vi "CRISValueRelay.vi"() -> ()   [LabVIEW 2013]
panel:
  in  "WL OOR":bool
  in  "PSB Cycle Number":i32
  in  "Linewidth Readout":dbl
  in  "Power Readout":dbl
  out "WS7 Pattern2 Data":dbl[](graph)
  out "Scan Number":i32
  in  "RILIS OK":bool
  out "CRIS OK":bool
  in  "Thin Readback":i32
  out "Thin Set":i32
  in  "Thick Readback":i32
  out "Thick Set":i32
  in  "Start supercycle":bool
  in  "Bunches in supercycle":i32
  in  "Bunches for HRS":i32
  in  "Power CRIS":dbl format="%#_10g"
  in  "Wavenumber CRIS":dbl format="%#_7g"
  in  "Update Rate (milliseconds)":u32=10
  out "Loop Counter":i32
  in  "Stop Button":bool
  out "isNew":bool
  in  "isOK":bool
  out "waveSet":dbl format="%.4g"
  in  "waveReadback":dbl format="%.4g"
  # "\\\\PCCRIS6\\Narrow Band TiSa Scanner Shared Variables\\isOK"
  # "\\\\PCCRIS6\\Narrow Band TiSa Scanner Shared Variables\\isOK"
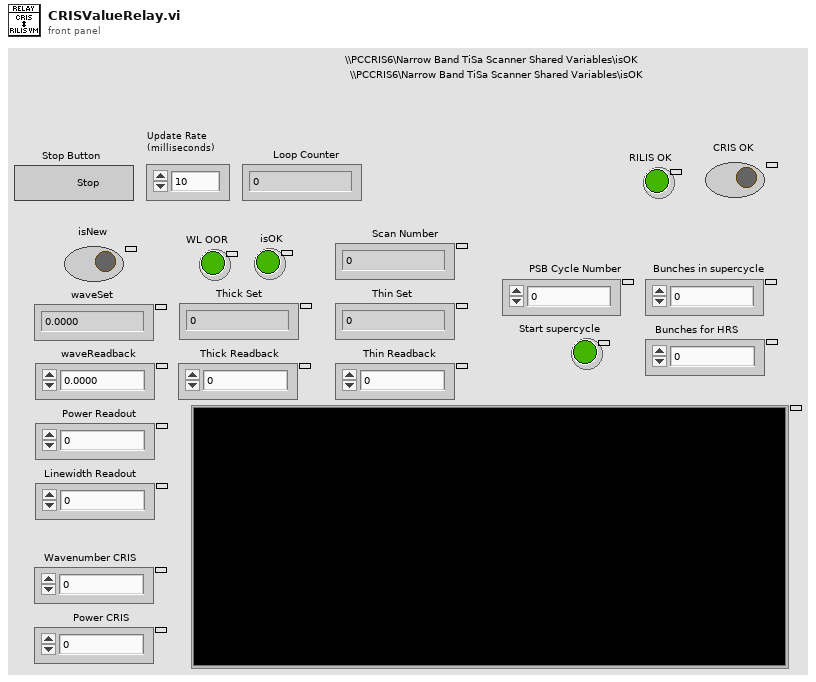
[diagram p1: front panel]
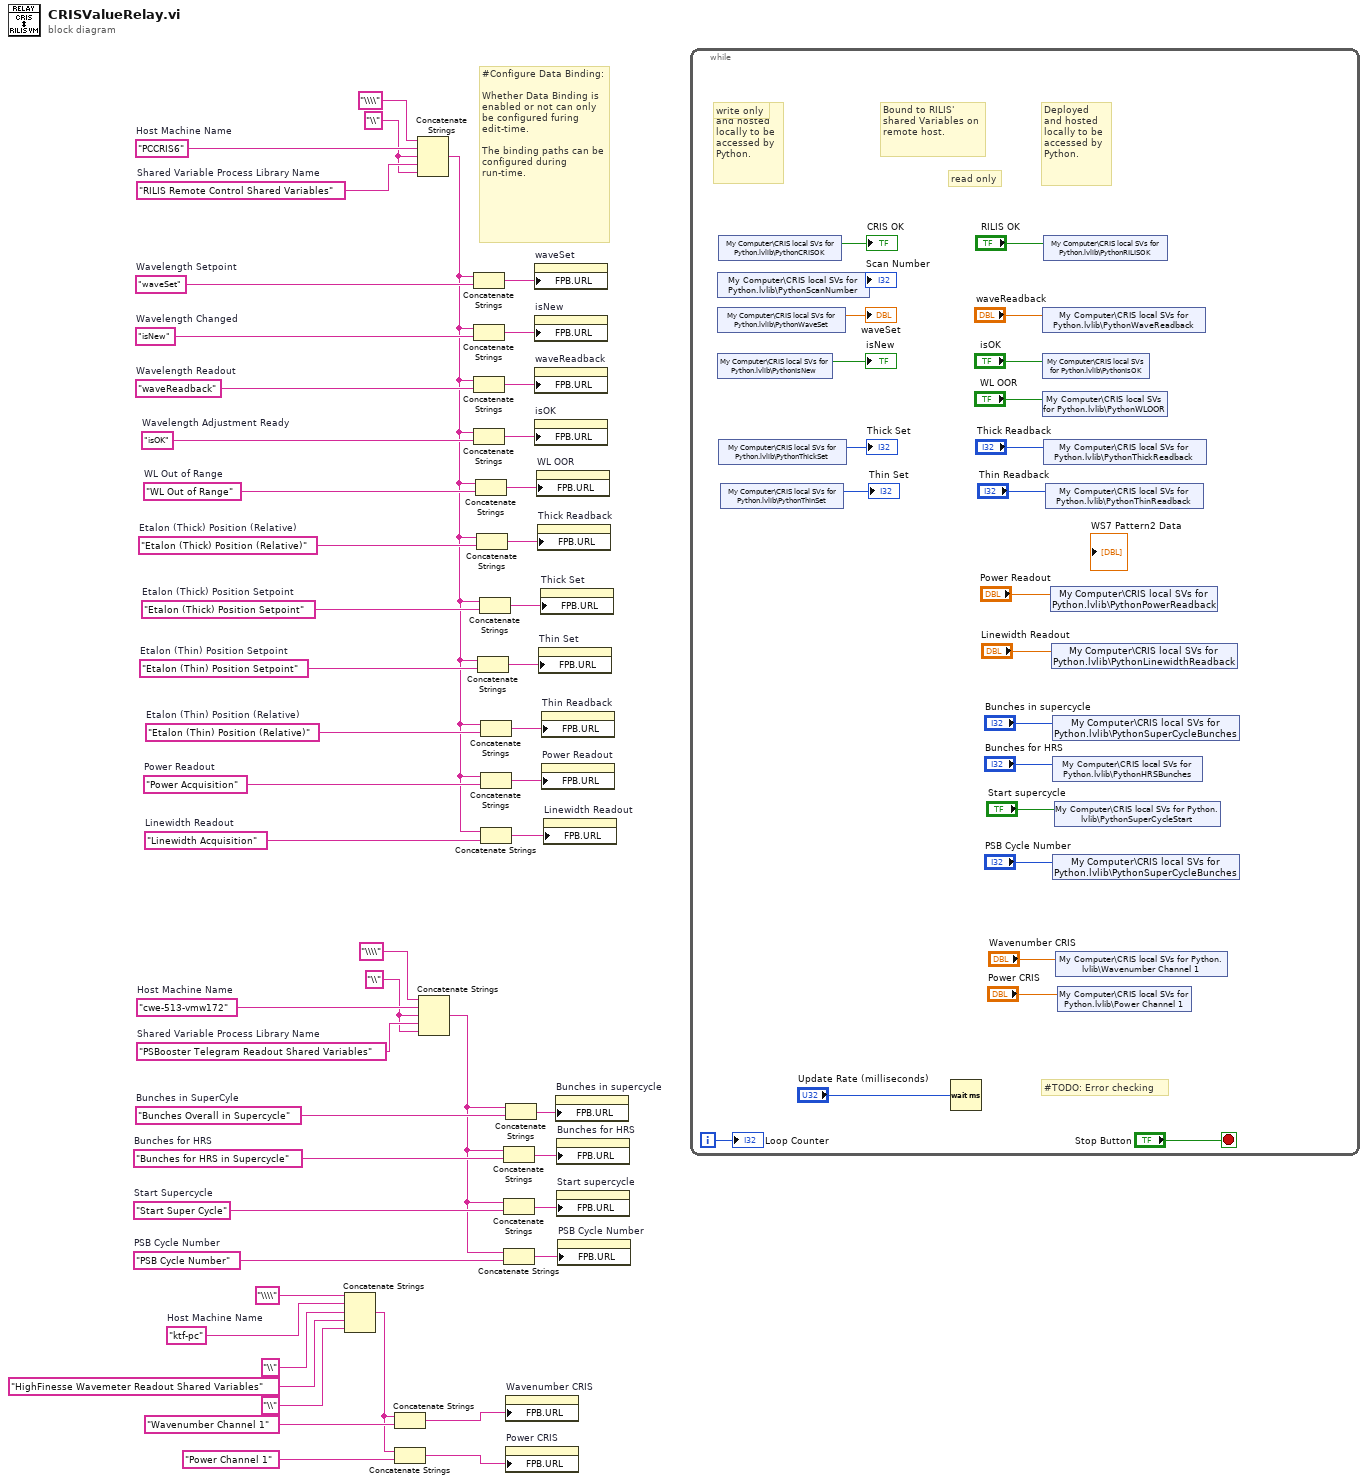
[diagram p0: block diagram]
diagram:
  w2 = "WL Out of Range"  # WL Out of Range
  w7 = "PSB Cycle Number"  # PSB Cycle Number
  w9 = "Linewidth Acquisition"  # Linewidth Readout
  w11 = "Power Acquisition"  # Power Readout
  w4 = "Etalon (Thin) Position Setpoint"  # Etalon (Thin) Position Setpoint
  w5 = "Etalon (Thin) Position (Relative)"  # Etalon (Thin) Position (Relative)
  w15 = "Etalon (Thick) Position Setpoint"  # Etalon (Thick) Position Setpoint
  w17 = "Etalon (Thick) Position (Relative)"  # Etalon (Thick) Position (Relative)
  w20 = "Start Super Cycle"  # Start Supercycle
  w22 = "Bunches Overall in Supercycle"  # Bunches in SuperCyle
  w23 = "\\"
  w24 = "PSBooster Telegram Readout Shared Variables"  # Shared Variable Process Library Name
  w25 = "cwe-513-vmw172"  # Host Machine Name
  w28 = "Bunches for HRS in Supercycle"  # Bunches for HRS
  w32 = "ktf-pc"  # Host Machine Name
  w47 = "\\"
  w46 = "waveSet"  # Wavelength Setpoint
  w40 = "waveReadback"  # Wavelength Readout
  w39 = "isOK"  # Wavelength Adjustment Ready
  w48 = "RILIS Remote Control Shared Variables"  # Shared Variable Process Library Name
  w41 = "isNew"  # Wavelength Changed
  w49 = "PCCRIS6"  # Host Machine Name
  # "#Configure Data Binding:\n\nWhether Data Binding is enabled or not can only be configured furing edit-time.\n\nThe binding paths can be configured during run-time."
  n1 = Concatenate Strings("\\\\", w32, "\\", "HighFinesse Wavemeter Readout Shared Variables", "\\") -> (w29:string)
  n2 = Concatenate Strings(w29, "Wavenumber Channel 1") -> (w31:string)
  n3 = Concatenate Strings(w29, "Power Channel 1") -> (w30:string)
  n4 = Concatenate Strings("\\\\", w49, w47, w48, w47) -> (w1:string)
  n5 = Concatenate Strings("\\\\", w25, w23, w24, w23) -> (w6:string)
  n6 = Concatenate Strings(w1, w46) -> (w45:string)
  n7 = Concatenate Strings(w1, w41) -> (w44:string)
  n8 = Concatenate Strings(w1, w40) -> (w43:string)
  n9 = Concatenate Strings(w1, w39) -> (w42:string)
  n10 = Concatenate Strings(w1, w2) -> (w3:string)
  n11 = Concatenate Strings(w1, w17) -> (w18:string)
  n12 = Concatenate Strings(w1, w4) -> (w14:string)
  n13 = Concatenate Strings(w1, w15) -> (w16:string)
  n14 = Concatenate Strings(w1, w5) -> (w13:string)
  n15 = Concatenate Strings(w1, w11) -> (w12:string)
  n16 = Concatenate Strings(w1, w9) -> (w10:string)
  n17 = Concatenate Strings(w6, w28) -> (w27:string)
  n18 = Concatenate Strings(w6, w20) -> (w19:string)
  n19 = Concatenate Strings(w6, w7) -> (w8:string)
  n20 = Concatenate Strings(w6, w22) -> (w21:string)
  n21 = property on="Wavenumber CRIS" class="DigNum (strict)"("FPB.URL"=w31) -> ()  [unwired: 2 in, 2 out]
  n22 = property on="Power CRIS" class="DigNum (strict)"("FPB.URL"=w30) -> ()  [unwired: 2 in, 2 out]
  n23 = property on="waveSet" class="DigNum (strict)"("FPB.URL"=w45) -> ()  [unwired: 2 in, 2 out]
  n24 = property on="isNew" class="Bool (strict)"("FPB.URL"=w44) -> ()  [unwired: 2 in, 2 out]
  n25 = property on="waveReadback" class="DigNum (strict)"("FPB.URL"=w43) -> ()  [unwired: 2 in, 2 out]
  n26 = property on="isOK" class="Bool (strict)"("FPB.URL"=w42) -> ()  [unwired: 2 in, 2 out]
  n27 = property on="WL OOR" class="Bool (strict)"("FPB.URL"=w3) -> ()  [unwired: 2 in, 2 out]
  n28 = property on="Thick Readback" class="DigNum (strict)"("FPB.URL"=w18) -> ()  [unwired: 2 in, 2 out]
  n29 = property on="Thin Set" class="DigNum (strict)"("FPB.URL"=w14) -> ()  [unwired: 2 in, 2 out]
  n30 = property on="Thick Set" class="DigNum (strict)"("FPB.URL"=w16) -> ()  [unwired: 2 in, 2 out]
  n31 = property on="Thin Readback" class="DigNum (strict)"("FPB.URL"=w13) -> ()  [unwired: 2 in, 2 out]
  n32 = property on="Power Readout" class="DigNum (strict)"("FPB.URL"=w12) -> ()  [unwired: 2 in, 2 out]
  n33 = property on="Linewidth Readout" class="DigNum (strict)"("FPB.URL"=w10) -> ()  [unwired: 2 in, 2 out]
  n34 = property on="Bunches in supercycle" class="DigNum (strict)"("FPB.URL"=w21) -> ()  [unwired: 2 in, 2 out]
  n35 = property on="Bunches for HRS" class="DigNum (strict)"("FPB.URL"=w27) -> ()  [unwired: 2 in, 2 out]
  n36 = property on="Start supercycle" class="Bool (strict)"("FPB.URL"=w19) -> ()  [unwired: 2 in, 2 out]
  n37 = property on="PSB Cycle Number" class="DigNum (strict)"("FPB.URL"=w8) -> ()  [unwired: 2 in, 2 out]
  n38 = while {
    i -> [w72]
    stop <- "Stop Button" stop-if-true
    # "#TODO: Error checking"
    # "Deployed and hosted locally to be accessed by Python."
    # "Deployed and hosted locally to be accessed by Python."
    # "read only"
    # "write only"
    # "Bound to RILIS' shared Variables on remote host."
    n39 = shared-variable "My Computer\\CRIS local SVs for Python.lvlib\\PythonScanNumber"() -> (→"Scan Number":i32)  [unwired: 1 in, 1 out]
    n40 = shared-variable "My Computer\\CRIS local SVs for Python.lvlib\\PythonWaveSet"() -> (→"waveSet":dbl)  [unwired: 1 in, 1 out]
    n41 = shared-variable "My Computer\\CRIS local SVs for Python.lvlib\\PythonIsNew"() -> (→"isNew":bool)  [unwired: 1 in, 1 out]
    n42 = shared-variable "My Computer\\CRIS local SVs for Python.lvlib\\PythonCRISOK"() -> (→"CRIS OK":bool)  [unwired: 1 in, 1 out]
    n43 = shared-variable "My Computer\\CRIS local SVs for Python.lvlib\\PythonThickSet"() -> (→"Thick Set":i32)  [unwired: 1 in, 1 out]
    n44 = shared-variable "My Computer\\CRIS local SVs for Python.lvlib\\PythonThinSet"() -> (→"Thin Set":i32)  [unwired: 1 in, 1 out]
    n45 = Wait (ms)(milliseconds to wait="Update Rate (milliseconds)") -> ()  [unwired: 1 out]
    n46 = shared-variable "My Computer\\CRIS local SVs for Python.lvlib\\PythonWaveReadback"("waveReadback") -> ()  [unwired: 1 in, 1 out]
    n47 = shared-variable "My Computer\\CRIS local SVs for Python.lvlib\\PythonIsOK"("isOK") -> ()  [unwired: 1 in, 1 out]
    n48 = shared-variable "My Computer\\CRIS local SVs for Python.lvlib\\PythonWLOOR"("WL OOR") -> ()  [unwired: 1 in, 1 out]
    n49 = shared-variable "My Computer\\CRIS local SVs for Python.lvlib\\PythonRILISOK"("RILIS OK") -> ()  [unwired: 1 in, 1 out]
    n50 = shared-variable "My Computer\\CRIS local SVs for Python.lvlib\\PythonThickReadback"("Thick Readback") -> ()  [unwired: 1 in, 1 out]
    n51 = shared-variable "My Computer\\CRIS local SVs for Python.lvlib\\PythonThinReadback"("Thin Readback") -> ()  [unwired: 1 in, 1 out]
    n52 = shared-variable "My Computer\\CRIS local SVs for Python.lvlib\\PythonPowerReadback"("Power Readout") -> ()  [unwired: 1 in, 1 out]
    n53 = shared-variable "My Computer\\CRIS local SVs for Python.lvlib\\PythonLinewidthReadback"("Linewidth Readout") -> ()  [unwired: 1 in, 1 out]
    n54 = shared-variable "My Computer\\CRIS local SVs for Python.lvlib\\PythonSuperCycleBunches"("Bunches in supercycle") -> ()  [unwired: 1 in, 1 out]
    n55 = shared-variable "My Computer\\CRIS local SVs for Python.lvlib\\PythonHRSBunches"("Bunches for HRS") -> ()  [unwired: 1 in, 1 out]
    n56 = shared-variable "My Computer\\CRIS local SVs for Python.lvlib\\PythonSuperCycleBunches"("PSB Cycle Number") -> ()  [unwired: 1 in, 1 out]
    n57 = shared-variable "My Computer\\CRIS local SVs for Python.lvlib\\PythonSuperCycleStart"("Start supercycle") -> ()  [unwired: 1 in, 1 out]
    n58 = shared-variable "My Computer\\CRIS local SVs for Python.lvlib\\Wavenumber Channel 1"("Wavenumber CRIS") -> ()  [unwired: 1 in, 1 out]
    n59 = shared-variable "My Computer\\CRIS local SVs for Python.lvlib\\Power Channel 1"("Power CRIS") -> ()  [unwired: 1 in, 1 out]
    "Loop Counter" <- w72
  }
